vi "PowerDown.vi"(8 "error in (no error)":errorcluster, 9 "DxBoot0":string, 10 "DxSupply":string, 11 "SMU handle in":refnum<k15> caption="SMU Handle in") -> (0 "error out":errorcluster, 3 "SMU handle out":refnum<k15>)   [LabVIEW 2018]
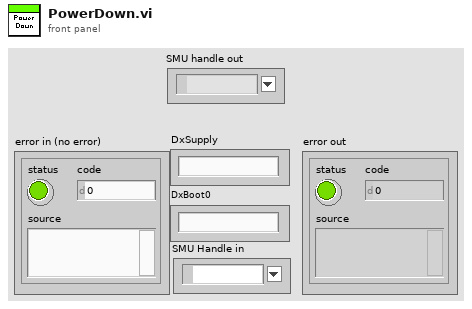
[diagram p1: front panel]
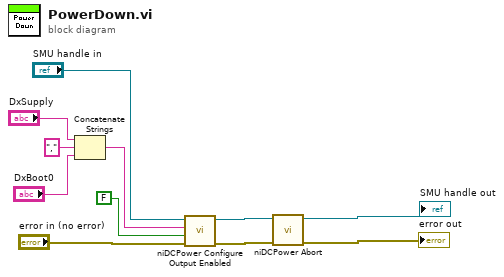
[diagram p0: block diagram]
diagram:
  n1 = Concatenate Strings("DxSupply", "," ("string"), "DxBoot0") -> (w8:string)
  n2 = call <instrlib>:"niDCPower Configure Output Enabled.vi"("error in (no error)"="error in (no error)", "output enabled"=FALSE, "channel name"=w8, "instrument handle"="SMU handle in") -> ("error out"=w2:errorcluster, "instrument handle out"=w1:refnum<k15>)  [unwired: 6 out]
  n3 = call <instrlib>:"niDCPower Abort.vi"("error in (no error)"=w2, "instrument handle"=w1) -> ("error out"=→"error out":errorcluster, "instrument handle out"=→"SMU handle out":refnum<k15>)  [unwired: 8 in]
